vi "Store Multicarrier CDMA2000 Forward State.vi"(0 "VISA Resource Name":refnum<visa-resource-name>, 5 "File Name (CDMA_DATA)":string="CDMA_DATA", 11 "error in (no error)":errorcluster {"code" format="%.0x"}) -> (4 "VISA Resource Name Out":refnum<visa-resource-name>, 15 "error out":errorcluster {"code" format="%.0x"})   [LabVIEW 2014, in "Agilent ESG Series.lvlib"]
doc: "This VI is used to store the current multicarrier custom CDMA2000 forward state into a designated file name.\nAfterward, you can recall this custom state from the instrument's memory with the Config CDMA2000 Forward.vi. - Forward Select - Multicarrier and Multicarrier - CUSTOM\n\nThis VI is valid only on instruments E44xxB with the 101 option or on instrument E4438C with option 401."
uses:
  Agilent ESG Series.lvlib
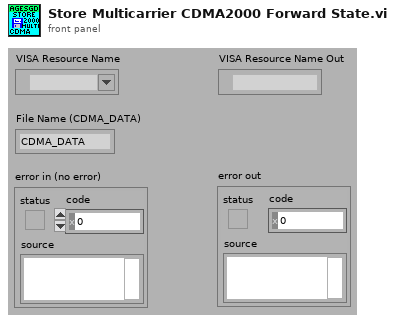
[diagram p1: front panel]
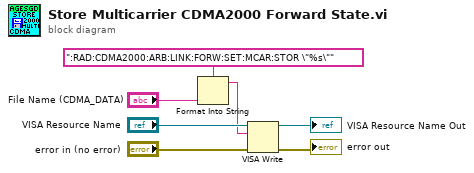
[diagram p0: block diagram]
diagram:
  n1 = Format Into String(format string=":RAD:CDMA2000:ARB:LINK:FORW:SET:MCAR:STOR \"%s\"", "File Name (CDMA_DATA)") -> (resulting string=w5:string)  [unwired: 2 in, 1 out]
  n2 = VISA Write(VISA resource name="VISA Resource Name", write buffer=w5, error in (no error)="error in (no error)") -> (VISA resource name out=→"VISA Resource Name Out":refnum<visa-resource-name>, error out=→"error out":errorcluster)  [unwired: 1 out]
